vi "hourSt.vi"() -> ()   [LabVIEW 2014, in "Sample.lvlib"]
uses:
  Sample.lvlib
panel:
  in  "HourSt":string(combo)
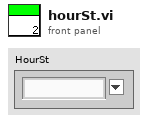
[diagram p1: front panel]
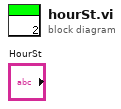
[diagram p0: block diagram]
diagram:
